vi "TC10 Status at Value Change.vi"(7 "NewVal":bool, 8 "error in":errorcluster, 10 "Interface Name String":string, 11 "XNET Refnum in":refnum<k21>) -> (0 "error out":errorcluster, 2 "Status Message String":string, 3 "XNET Refnum out":refnum<k21>)   [LabVIEW 2025, in "Automotive Ethernet Bus Monitor UI.lvlib"]
doc: "Setting TC10 to sleep or awake depending of the NewVal."
uses:
  Automotive Ethernet Bus Monitor UI.lvlib
  <vilib>/xnet/xnet.llb/XNET Write (State Ethernet Wake).vi
  <vilib>/xnet/xnet.llb/XNET Write (State Ethernet Sleep).vi
  <resource>/objmgr/xnet.rc
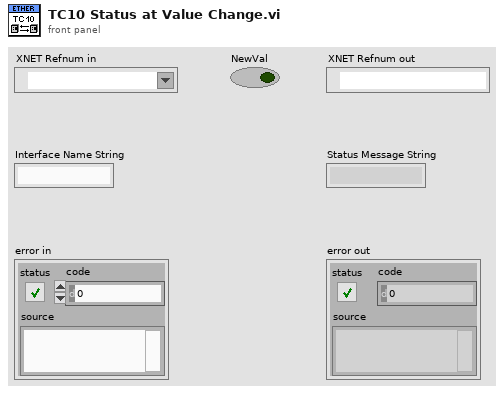
[diagram p1: front panel]
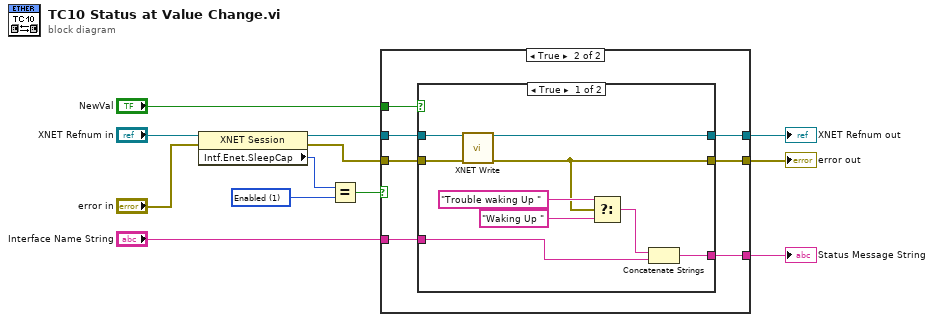
[diagram p0: block diagram]
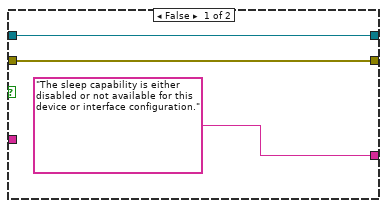
[diagram p2: hidden frame]
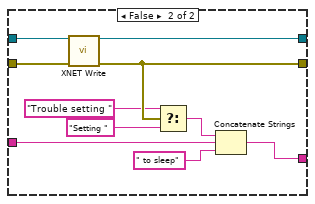
[diagram p3: hidden frame]
diagram:
  w2 = u32 1 items=["Disabled / Not Available", "Enabled"] ("Interface:Ethernet:Sleep Capability")
  n1 = property class="XNET Session"(reference="XNET Refnum in", error in="error in") -> (reference out=w6:refnum<k21>, error out=w5:errorcluster, "Intf.Enet.SleepCap"=w1:u32)
  n2 = Equal?(x=w1, y=w2) -> (x = y?=w3:bool)
  n3 = case shown="True" w3 {
    tunnel: "NewVal" -> [_ w22]
    tunnel: w5 -> [w15 w21]
    tunnel: w6 -> [w14 w20]
    tunnel: [w14 w19] -> w11
    tunnel: [w15 w18] -> w10
    tunnel: "Interface Name String" -> [_ w17]
    tunnel: ["The sleep capability is either disabled or not available for this device or interface configuration." w16] -> w12
    frame False {
    }
    frame True {
      n4 = case shown="True" w22 {
        tunnel: w21 -> [w31 w41]
        tunnel: w20 -> [w30 w40]
        tunnel: [w29 w39] -> w19
        tunnel: [w24 w38] -> w18
        tunnel: w17 -> [w28 w37]
        tunnel: [w23 w32] -> w16
        frame True {
          n5 = call-poly <vilib>:"XNET Write.vi"("session in"=w30, "error in (no error)"=w31) -> ("session out"=w29:refnum<k21>, "error out"=w24:errorcluster)  [unwired: 12 in]
          n6 = Select(t="Trouble waking Up ", s=w24, f="Waking Up ") -> (s? t:f=w25:string)
          n7 = Concatenate Strings(w25, w28) -> (w23:string)
        }
        frame False {
          n8 = call-poly <vilib>:"XNET Write.vi"("session in"=w40, "error in (no error)"=w41) -> ("session out"=w39:refnum<k21>, "error out"=w38:errorcluster)  [unwired: 12 in]
          n9 = Select(t="Trouble setting ", s=w38, f="Setting ") -> (s? t:f=w35:string)
          n10 = Concatenate Strings(w35, w37, " to sleep" ("string")) -> (w32:string)
        }
      }
    }
  }
  "Status Message String" <- w12
  "XNET Refnum out" <- w11
  "error out" <- w10
